vi "LabVIEW File_ Health Monitoring System.vi"() -> ()   [LabVIEW 2020]
panel:
  in  "PORT NAME":refnum<visa-resource-name>
  in  "Data of patient":string[][](table)
  out "Temperature":dbl(graph)
  out "Heart rate BPM":dbl(graph)
  out "Temperature":dbl(slide) scale=0.0..100.0
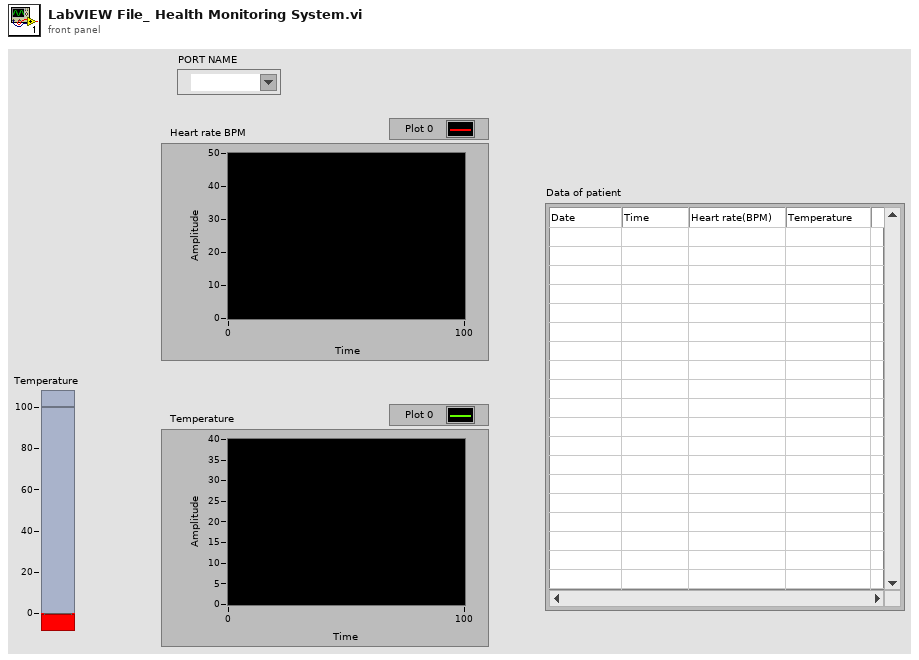
[diagram p1: front panel]
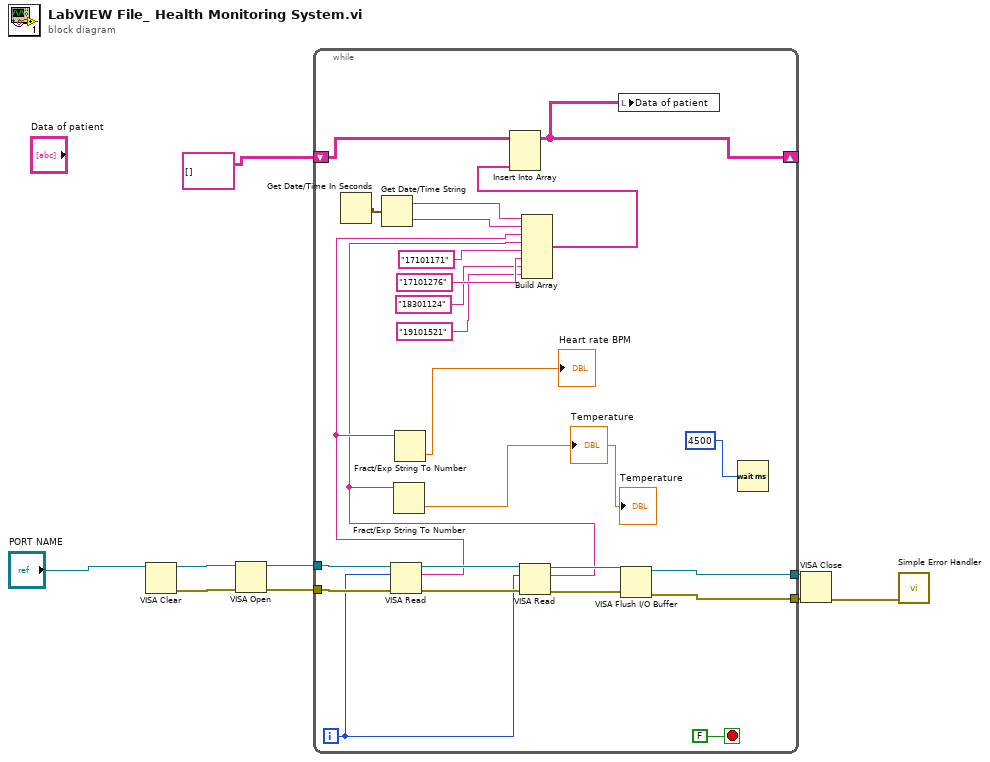
[diagram p0: block diagram]
diagram:
  n1 = VISA Clear(VISA resource name="PORT NAME") -> (VISA resource name out=w8:refnum<visa-resource-name>, error out=w9:errorcluster)  [unwired: 1 in]
  n2 = VISA Open(error in (no error)=w9, VISA resource name=w8) -> (VISA resource name=w6:refnum<visa-resource-name>, error out=w5:errorcluster)  [unwired: 3 in]
  n3 = while {
    tunnel: w6 -> [w34]
    tunnel: w5 -> [w33]
    tunnel: [w30] -> w4
    tunnel: [w29] -> w3
    shift-right: [w23] -> _
    shift-left: string[][] [] -> [w24]
    i -> [w26]
    stop <- FALSE stop-if-true
    n4 = Get Date/Time In Seconds() -> (seconds since 1Jan1904=w22:timestamp)
    n5 = Get Date/Time String(seconds (now)=w22) -> (date string=w21:string, time string=w20:string)  [unwired: 2 in]
    n6 = VISA Read(VISA resource name=w34, byte count=w26, error in (no error)=w33) -> (VISA resource name out=w32:refnum<visa-resource-name>, read buffer=w19:string, error out=w28:errorcluster)  [unwired: 1 out]
    n7 = Fract/Exp String To Number(string=w19) -> (number=→"Heart rate BPM":dbl)  [unwired: 3 in, 1 out]
    n8 = VISA Read(VISA resource name=w32, byte count=w26, error in (no error)=w28) -> (VISA resource name out=w31:refnum<visa-resource-name>, read buffer=w18:string, error out=w27:errorcluster)  [unwired: 1 out]
    n9 = Fract/Exp String To Number(string=w18) -> (number=→"Temperature" →"Temperature":dbl)  [unwired: 3 in, 1 out]
    n10 = Build Array "Build Array"(w21, w20, w19, w18, "17101171", "17101276", "18301124", "19101521") -> (w17:string[])
    n11 = Insert Into Array "Insert Into Array"(array=w24, new element=w17) -> (w23:string[][])  [unwired: 2 in]
    n12 = local write "Data of patient"(w23) -> ()
    n13 = VISA Flush I/O Buffer(VISA resource name=w31, error in (no error)=w27) -> (VISA resource name out=w30:refnum<visa-resource-name>, error out=w29:errorcluster)  [unwired: 1 in]
    n14 = Wait (ms)(milliseconds to wait=u32 4500 ("millisecond timer value")) -> ()  [unwired: 1 out]
  }
  n15 = VISA Close(VISA resource name=w4, error in (no error)=w3) -> (error out=w7:errorcluster)
  n16 = call <vilib>:"Simple Error Handler.vi"("error in (no error)"=w7) -> ()  [unwired: 4 in, 5 out]
